vi "Meas Result Generate TWM Digitizer Correction.vi"(8 "error in":errorcluster, 11 "meas":T5={"swp cfg"={"N"=0, "R"=0, "f list"=[], "smpl delay"=0.0, "set delay"=0.0, "set delay np"=0.0, "meas root"=path "", "meas name"="", "meas a-index"=FALSE, "rnd sweep"=FALSE, "mode"=enum."Frequency", "swp mode"=enum."Linear", "avg"=0, "subrec"=0, "multi-freq"=FALSE, "selfcal"=FALSE, "selfcal period [h]"=0.0}, "bridge"={"type"=enum."TWM client", "TWM"={"pipe name"="", "parameters"=[], "handle"=0, "fixed aper [s]"=0.0, "f-list [Hz]"=[], "discrete f-list"=FALSE, "unc mode"=enum."None", "unc mcc"=0, "unc first"=FALSE, "alg id"=enum."TWM-LowZ - Low Z measurement"}, "last f"=0.0, "bias comp"={"bias type"=enum."dummy", "VISA"="", "Enable"=FALSE, "channel qu"=[], "channel Uinit"=[]}, "sim mode"=enum."Generic RLC network", "channel idns"=[], "sim phases"=1}, "src"={"type"=enum."Tektronix AFG3101C", "afg"={"VISA"="", "const"=0.0, "gen DC"=FALSE, "ext ref"=FALSE}, "cDAQ dds"={"device"="", "channels"=[], "mclk source"="", "mclk [Hz]"=0.0, "fs [Hz]"=0.0, "block [s]"=0.0, "buf [s]"=0.0, "task"="", "cmd queue"=refnum, "proc ref"=refnum, "smpl clock out"="/cDAQ3/PFI0", "export smpl clock"=FALSE, "DC ofs [V]"=[], "timebase source"="", "timebase mode"=enum."Local", "dither"=enum."Disabled", "dither level"=0.0, "phase [rad]"=[]}, "gain [V/A]"=1.0, "F5xxx session"={"VISA"="", "mode"=enum."AC voltage", "Earth on"=FALSE, "Ext ref lock"=FALSE}, "t3awg"={"VISA"="", "use ext ref"=FALSE, "ext ref [Hz]"=0.0, "load Z"=enum."High Z", "ramdac max n"=0, "noise dither [V]"=0.0, "t3awg fs rules"=[], "channels"=0, "ramdac min n"=0}}, "results"=refnum, "dvm"={"type"=enum."Disabled", "F5790"={"VISA"="", "Input"=enum."input 1", "Digital filter restart"=enum."medium", "hi resolution"=enum."off", "Digital filter mode"=enum."off", "ext guard"=FALSE}}, "thermo"={"type"=enum."COMET Tx5xx (ethernet)", "comment"="", "tag"="", "refresh"=5.0, "IP"="", "port"=502, "VISA"="", "last readout"=timestamp(0 s since 1904-01-01), "TCP ref"=refnum, "VISA sess"="", "idn"="", "press"=0.0, "RH"=0.0, "temp"=0.0, "pres cor"=[], "RH cor"=[], "temp cor"=[], "try left"=0, "failed"=FALSE, "RTD set"=[], "RTD inv"=[], "range"=0.0, "net mode"=enum."MODBUS", "try fail"=enum."Stop trying - return NaN", "timeout [s]"=0.0, "max retries"=0, "sim t [deg]"=0.0, "status"=0}} {"thermo"."status" items=["ok", "retry", "failed"]; "thermo"."RTD inv" format="%.1f"; "thermo"."RTD set" format="%.1f"; "thermo"."temp cor" format="%.1f"; "thermo"."RH cor" format="%.1f"; "thermo"."pres cor" format="%.1f"; "thermo"."refresh" min=0.1 max=1000.0 format="%.2f"; "src"."t3awg"."t3awg fs rules"."fs-step [Hz]" format="%#_6p"; "src"."t3awg"."t3awg fs rules"."fs-max [Hz]" format="%#_6p"; "src"."t3awg"."t3awg fs rules"."for f0 <" format="%#_6p"; "src"."t3awg"."t3awg fs rules"."fs-min [Hz]" format="%#_6p"; "src"."cDAQ dds"."channels" min=0 step=1; "bridge"."TWM"."f-list [Hz]" format="%#_6p"; "swp cfg"."f list"."bias" format="%#_3p"; "swp cfg"."f list"."level" format="%#_3p"; "swp cfg"."f list"."fs [Hz]" format="%#_5p"; "swp cfg"."f list"."time [s]" format="%#_3p"; "swp cfg"."f list"."f/fs" format="%#_3p"; "swp cfg"."f list"."periods" format="%#_3f"; "swp cfg"."f list"."f [Hz]" format="%#_5p"}) -> (0 "error out":errorcluster)   [LabVIEW 2020]
doc: "Generates simple TWM digitizer correction from measured data."
uses:
  meas session.ctl
  Meas Sweep Config.ctl
  Meas Freq Info.ctl
  meas_swp_mode.ctl
  meas_sweep_flist_mode.ctl
  bridge/Bridge Session.ctl
  bridge/Bridge Type.ctl
  drivers/TWM client/TWM Session.ctl
  drivers/TWM client/TWM parameters.ctl
  drivers/TWM client/Meas Proc QWTB Uncertainty Mode.ctl
  bridge/Bridge Algorithm.ctl
  bridge/Bridge Bias Session.ctl
  bridge/Bridge Bias Type.ctl
  bridge/Bridge Sim Mode.ctl
  source/Source Session.ctl
  source/Source Type.ctl
  drivers/AFG3101C/AFG3101C Session.ctl
  drivers/cDAQ DDS/cDAQ DDS Session.ctl
  drivers/cDAQ DDS/cDAQ DDS Setup.ctl
  drivers/cDAQ DDS/cDAQ DDS Timebase Mode.ctl
  drivers/cDAQ DDS/cDAQ DDS Dither.ctl
  drivers/Fluke 5XXX/top_lev/F5xxx_session.ctl
  drivers/Fluke 5XXX/top_lev/F5xxx_output_mode.ctl
  drivers/T3AWG3K/toplevel/T3AWG Session.ctl
  drivers/T3AWG3K/toplevel/T3AWG Load Z.ctl
  drivers/T3AWG3K/toplevel/fgen_ramdac_fs_rules.ctl
  results/Meas Results Ref.ctl
  results/Meas Results.ctl
  bridge/Bridge Frequency Readings Data.ctl
  drivers/TWM client/Meas Proc QWTB Spectrum Data.ctl
  drivers/TWM client/TWM Phase Info.ctl
  dvm/dvm session.ctl
  dvm/dvm type.ctl
  drivers/Fluke 5790A/top_level/F5790 session.ctl
  thermo/thermo.ctl
  thermo/thermo_types.ctl
  thermo/Thermometer Fail Action.ctl
  results/Meas Results Correction Structuring Mode.ctl
  Meas Results TWM Digitizer Correction Data.ctl
  Meas Results TWM Correction Digitizer Type.ctl
  Meas Results TWM InpZ Correction Uncertainty Config.ctl
  drivers/T3AWG3K/Active Technologies AWG3000.lvlib
panel:
  in  "u(Gp) [S]":dbl
  in  "u(Cp) [%]":dbl
  in  "u(Gp) [%]":dbl
  in  "u(Cp) [F]":dbl
  out "alg id":T1 caption="bridge.TWM.alg id"
  in  "Digitizer type":T2=enum."HP3458A"
  in  "Estimate non-linearity":bool
  in  "btn exit":bool
  out "last path":path
  out "correction data":T3
  in  "Use aperture correction":bool=TRUE
  in  "Use time shift":bool=TRUE
  in  "Mode":T4
  in  "btn export":bool
  out "table":string[][](table) caption="Overview"
  # "Uncertainty:"
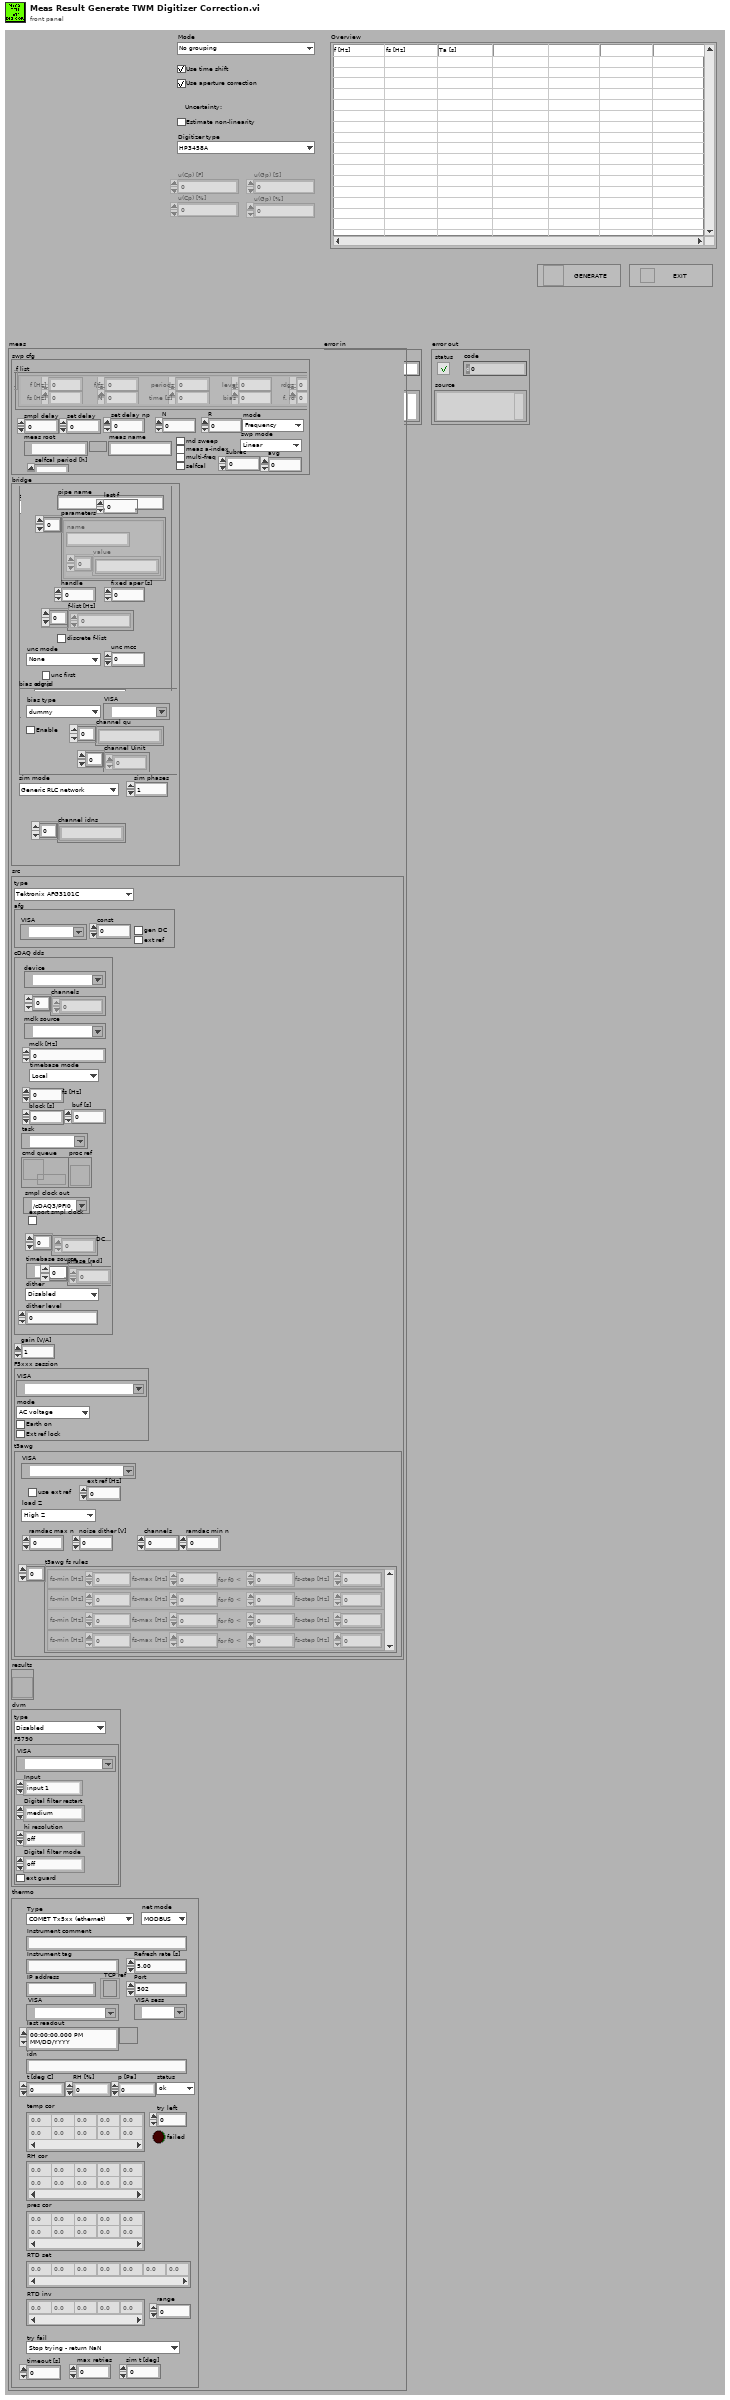
[diagram p1: front panel]
types:
  T1 = typedef "Bridge Algorithm.ctl" = enum16{"TWM-LowZ - Low Z measurement", "TWM-InpZ - Digitizer input Z measurement", "TWM-TIAZ - High Z using TIA"}
  T2 = typedef "Meas Results TWM Correction Digitizer Type.ctl" = enum16{"Unknown", "HP3458A", "NI9238"}
  T3 = typedef "Meas Results TWM Digitizer Correction Data.ctl" = cluster{"gains [V/V]":dbl[][][], "phases [rad]":dbl[][][], "timeshifts [s]":dbl[][], "f [Hz]":dbl[], "fs list [Hz]":dbl[], "aperture list [s]":dbl[], "channels":string[], "Mode":T4, "aperture correction":bool, "ranges [V]":dbl[], "amp [V]":dbl[][], "apertures [s]":dbl[], "unc gains [V/V]":dbl[][][], "unc phases [rad]":dbl[][][]}
  T4 = typedef "Meas Results Correction Structuring Mode.ctl" = enum16{"No grouping", "Group by apertures (3458A)", "Group by fs (generic digitizer)"}
  T5 = typedef "meas session.ctl" = cluster{"swp cfg":T6, "bridge":T10, "src":T18, "results":T29, "dvm":T30, "thermo":T33}
  T6 = typedef "Meas Sweep Config.ctl" = cluster{"N":i32, "R":i32, "f list":T7[], "smpl delay":dbl, "set delay":dbl, "set delay np":dbl, "meas root":path, "meas name":string, "meas a-index":bool, "rnd sweep":bool, "mode":T8, "swp mode":T9, "avg":i32, "subrec":i32, "multi-freq":bool, "selfcal":bool, "selfcal period [h]":dbl}
  T7 = typedef "Meas Freq Info.ctl" = cluster{"f [Hz]":dbl, "periods":dbl, "f/fs":dbl, "time [s]":dbl, "fs [Hz]":dbl, "N":i32, "level":dbl, "bias":dbl, "rdgs":i32, "f. id":i32}
  T8 = typedef "meas_swp_mode.ctl" = enum16{"Frequency", "Level", "Bias"}
  T9 = typedef "meas_sweep_flist_mode.ctl" = enum16{"Linear", "Log10"}
  T10 = typedef "Bridge Session.ctl" = cluster{"type":T11, "TWM":T12, "last f":dbl, "bias comp":T15, "sim mode":T17, "channel idns":string[], "sim phases":i32}
  T11 = typedef "Bridge Type.ctl" = enum16{"TWM client", "dummy"}
  T12 = typedef "TWM Session.ctl" = cluster{"pipe name":string, "parameters":T13[], "handle":i32, "fixed aper [s]":dbl, "f-list [Hz]":dbl[], "discrete f-list":bool, "unc mode":T14, "unc mcc":i32, "unc first":bool, "alg id":T1}
  T13 = typedef "TWM parameters.ctl" = cluster{"name":string, "value":string[]}
  T14 = typedef "Meas Proc QWTB Uncertainty Mode.ctl" = enum16{"None", "GUF", "Monte Carlo"}
  T15 = typedef "Bridge Bias Session.ctl" = cluster{"bias type":T16, "VISA":refnum<visa-resource-name>, "Enable":bool, "channel qu":string[], "channel Uinit":dbl[]}
  T16 = typedef "Bridge Bias Type.ctl" = enum16{"dummy", "CMI LiBbias V1.0"}
  T17 = typedef "Bridge Sim Mode.ctl" = enum16{"Generic RLC network", "Interchannel transfer", "Input impedance"}
  T18 = typedef "Source Session.ctl" = cluster{"type":T19, "afg":T20, "cDAQ dds":T21, "gain [V/A]":dbl, "F5xxx session":T24, "t3awg":T26}
  T19 = typedef "Source Type.ctl" = enum16{"Tektronix AFG3101C", "cDAQ DAC", "Fluke 5xxx", "Agilent 33120A", "R&S SMT", "Teledyne LeCroy T3AWG", "dummy"}
  T20 = typedef "AFG3101C Session.ctl" = cluster{"VISA":refnum<visa-resource-name>, "const":dbl, "gen DC":bool, "ext ref":bool}
  T21 = typedef "cDAQ DDS Session.ctl" = cluster{"device":tag, "channels":i32[], "mclk source":tag, "mclk [Hz]":dbl, "fs [Hz]":dbl, "block [s]":dbl, "buf [s]":dbl, "task":refnum<k21>, "cmd queue":refnum<queue>, "proc ref":refnum<vi>, "smpl clock out":tag, "export smpl clock":bool, "DC ofs [V]":dbl[], "timebase source":tag, "timebase mode":T22, "dither":T23, "dither level":dbl, "phase [rad]":dbl[]}
  T22 = typedef "cDAQ DDS Timebase Mode.ctl" = enum16{"Local", "Take from ADC (e.g. NI 9238)", "Other source"}
  T23 = typedef "cDAQ DDS Dither.ctl" = enum16{"Disabled", "Gaussian"}
  T24 = typedef "F5xxx_session.ctl" = cluster{"VISA":refnum<visa-resource-name>, "mode":T25, "Earth on":bool, "Ext ref lock":bool}
  T25 = typedef "F5xxx_output_mode.ctl" = enum16{"AC voltage", "AC current"}
  T26 = typedef "Active Technologies AWG3000.lvlib/T3AWG Session.ctl" = cluster{"VISA":refnum<visa-resource-name>, "use ext ref":bool, "ext ref [Hz]":dbl, "load Z":T27, "ramdac max n":i32, "noise dither [V]":dbl, "t3awg fs rules":T28[], "channels":i32, "ramdac min n":i32}
  T27 = typedef "Active Technologies AWG3000.lvlib/T3AWG Load Z.ctl" = enum16{"High Z", "50 Ohm"}
  T28 = typedef "Active Technologies AWG3000.lvlib/fgen_ramdac_fs_rules.ctl" = cluster{"fs-min [Hz]":dbl, "fs-max [Hz]":dbl, "for f0 < ":dbl, "fs-step [Hz]":dbl}
  T29 = typedef "Meas Results Ref.ctl" = refnum<vi>
  T30 = typedef "dvm session.ctl" = cluster{"type":T31, "F5790":T32}
  T31 = typedef "dvm type.ctl" = enum16{"Disabled", "Simulated", "Fluke 5790A"}
  T32 = typedef "F5790 session.ctl" = cluster{"VISA":refnum<visa-resource-name>, "Input":enum16{"input 1", "input 2", "wide-band"}, "Digital filter restart":enum16{"medium", "fine", "coarse"}, "hi resolution":enum16{"off", "on"}, "Digital filter mode":enum16{"off", "fast", "medium", "slow"}, "ext guard":bool}
  T33 = typedef "thermo.ctl" = cluster{"type":T34, "comment":string, "tag":string, "refresh":dbl, "IP":string, "port":u16, "VISA":refnum<visa-resource-name>, "last readout":timestamp, "TCP ref":refnum<k5>, "VISA sess":refnum<visa-resource-name>, "idn":string, "press":dbl, "RH":dbl, "temp":dbl, "pres cor":dbl[][], "RH cor":dbl[][], "temp cor":dbl[][], "try left":i32, "failed":bool, "RTD set":dbl[], "RTD inv":dbl[], "range":dbl, "net mode":enum16{"MODBUS", "HTTP"}, "try fail":T35, "timeout [s]":dbl, "max retries":i32, "sim t [deg]":dbl, "status":u16}
  T34 = typedef "thermo_types.ctl" = enum16{"Disabled", "Simulated", "COMET Tx5xx (ethernet)", "Keithley 2002 (GPIB) + RTD", "Agilent 344xx (GPIB) + RTD"}
  T35 = typedef "Thermometer Fail Action.ctl" = enum16{"Stop trying - keep last value", "Stop trying - return NaN", "Generate error - stop sweep"}
  T36 = typedef "Meas Results TWM InpZ Correction Uncertainty Config.ctl" = cluster{"u(Cp) [F]":dbl, "u(Cp) [%]":dbl, "u(Gp) [S]":dbl, "u(Gp) [%]":dbl}
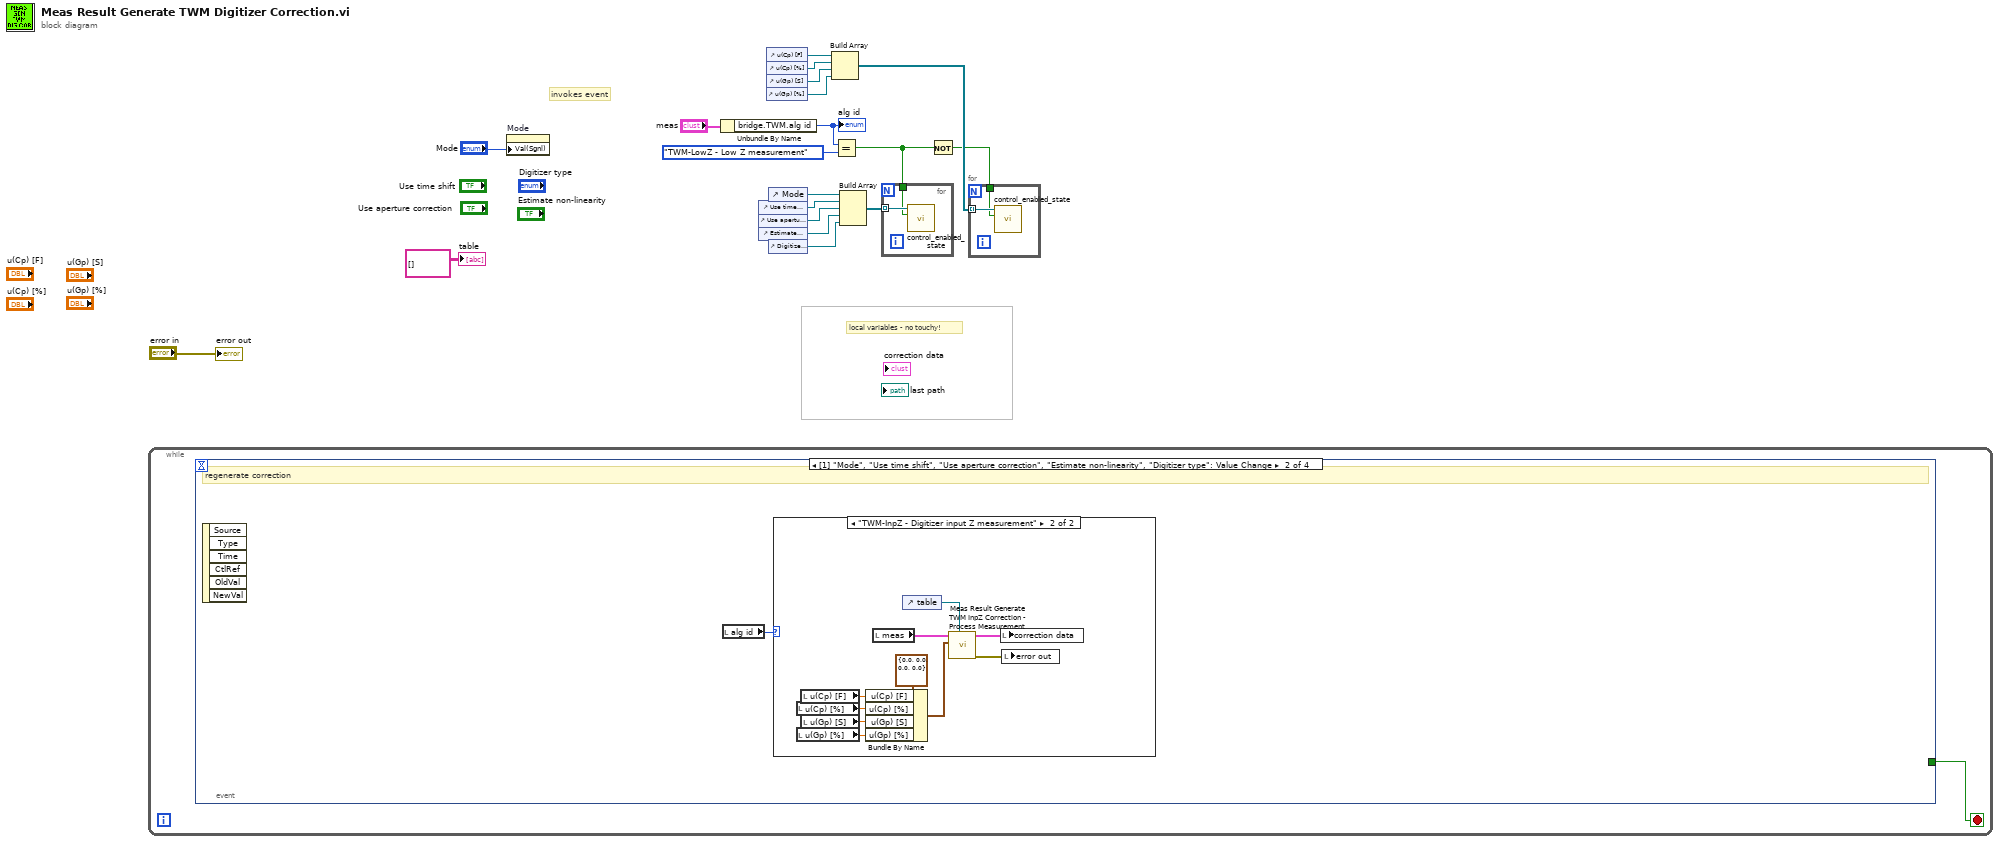
[diagram p0: block diagram]
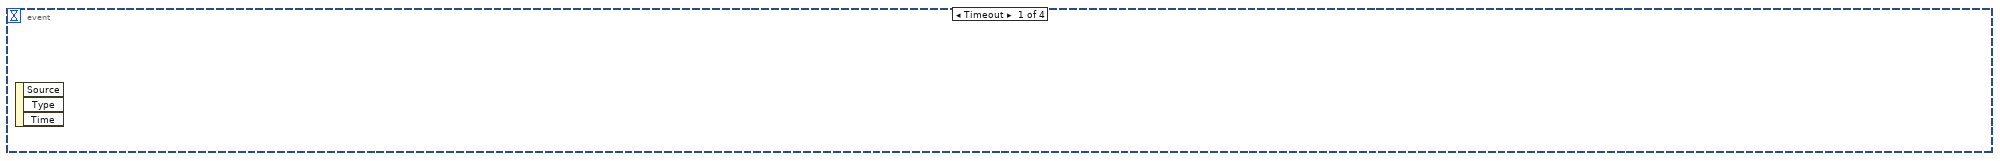
[diagram p2: hidden frame]
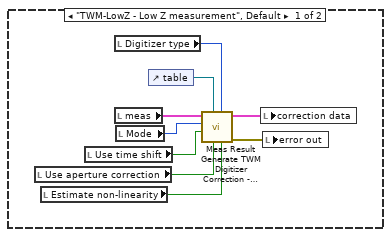
[diagram p3: hidden frame]
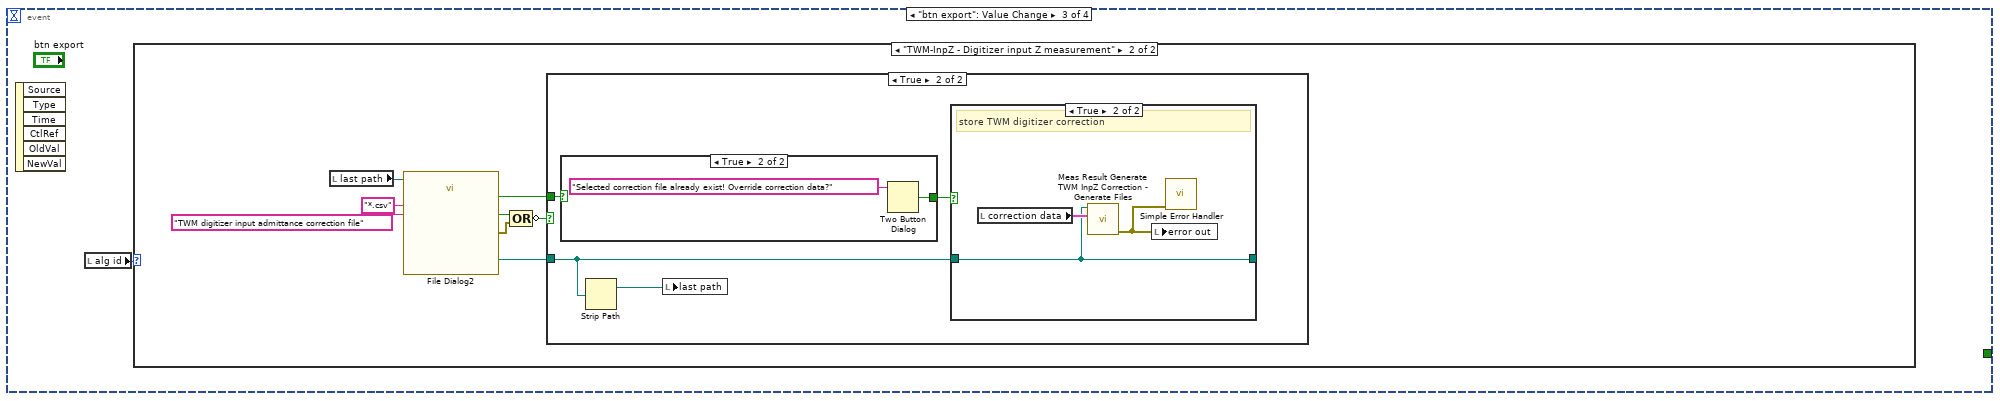
[diagram p4: hidden frame]
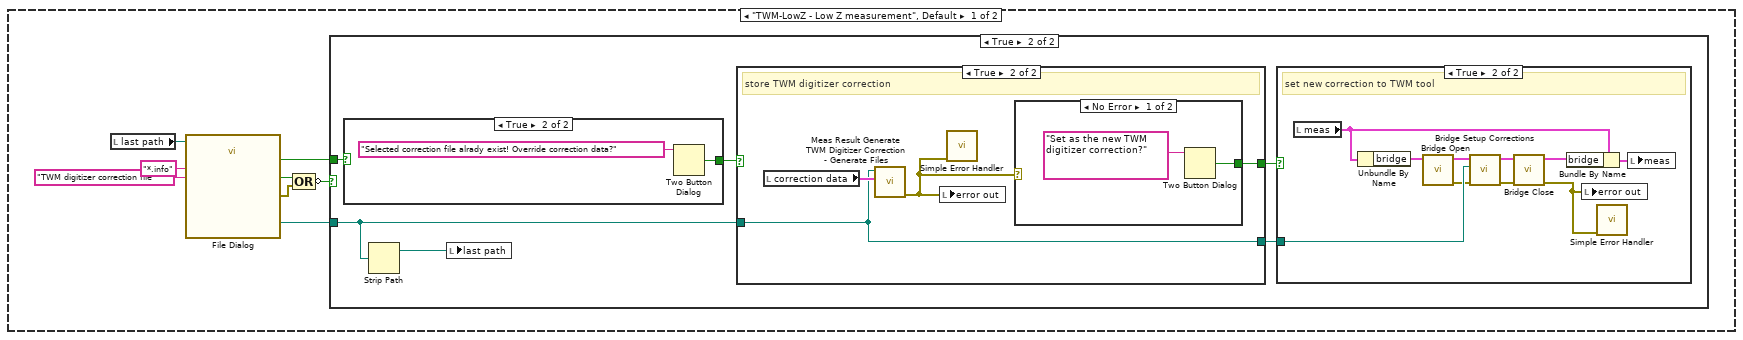
[diagram p5: hidden frame]
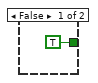
[diagram p8: hidden frame]
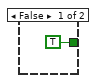
[diagram p12: hidden frame]
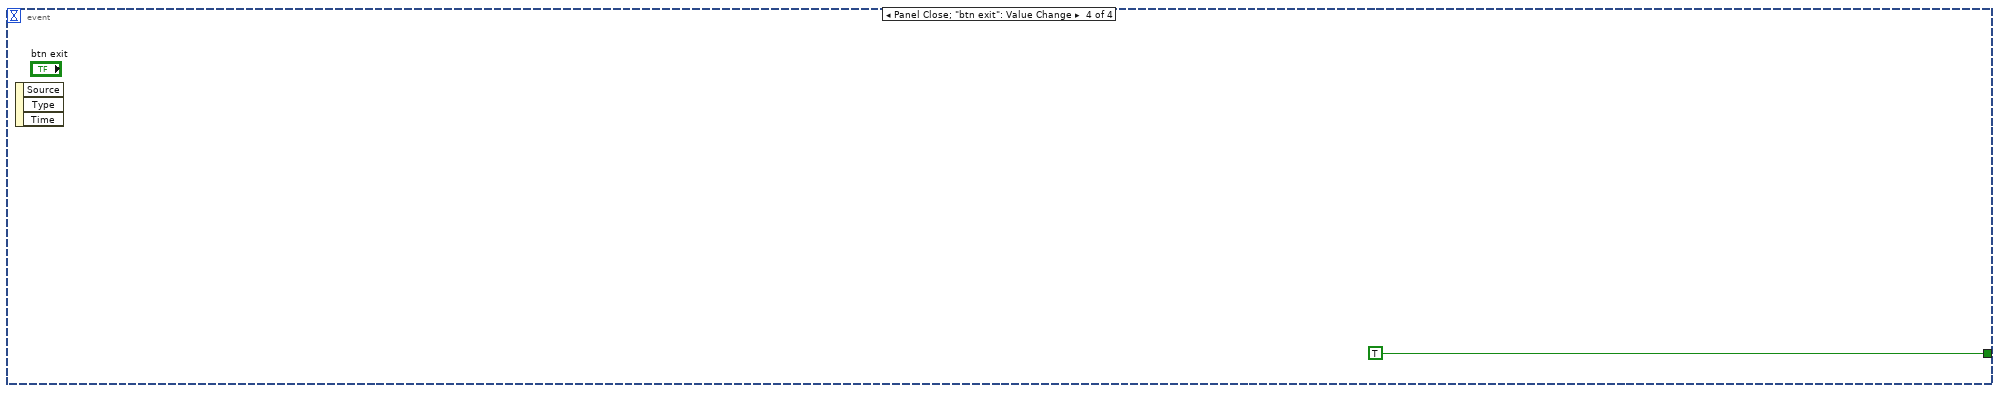
[diagram p14: hidden frame]
diagram:
  # "local variables - no touchy!"
  # "invokes event"
  n1 = while {
    stop <- w20 stop-if-true
    n2 = event shown="[1] \"Mode\", \"Use time shift\", \"Use aperture correction\", \"Estimate non-linearity\", \"Digitizer type\": Value Change" {
      selector: _ -> [_ _ _ _]
      dyn-events: _ -> [_ _ _ _]
      timeout: _ -> [_ _ _ _]
      tunnel: [_ _ _ TRUE] -> w20
      event Timeout {
        n3 = event-data() -> ()  [unwired: 1 in, 3 out]
      }
      event "Use time shift", "Use aperture correction", "Estimate non-linearity": Value Change {
        # "regenerate correction"
        n4 = event-data() -> ()  [unwired: 1 in, 6 out]
        n5 = local read "alg id"() -> (w21:T1)
        n6 = case shown="\"TWM-InpZ - Digitizer input Z measurement\"" w21 {
          frame "TWM-LowZ - Low Z measurement", Default {
            n7 = local read "Use aperture correction"() -> (w25:bool)
            n8 = local read "Estimate non-linearity"() -> (w23:bool)
            n9 = local read "Use time shift"() -> (w26:bool)
            n10 = local read "Digitizer type"() -> (w22:T2)
            n11 = local read "meas"() -> (w28:T5)
            n12 = local read "Mode"() -> (w27:T4)
            n13 = control-ref of="table"() -> (w29:refnum<vi>)
            n14 = call "Meas Result Generate TWM Digitizer Correction - Process Measurement.vi"("Estimate non-linearity (False)"=w23, "digitizer type"=w22, "use aperture correction (true)"=w25, "table ref"=w29, "use time shift (true)"=w26, "Mode"=w27, "meas"=w28) -> ("error out"=w30:errorcluster, "correction data"=w24:T3)  [unwired: 3 in]
            n15 = local write "correction data"(w24) -> ()
            n16 = local write "error out"(w30) -> ()
          }
          frame "TWM-InpZ - Digitizer input Z measurement" {
            n17 = local read "u(Cp) [%]"() -> (w33:dbl)
            n18 = local read "u(Gp) [%]"() -> (w36:dbl)
            n19 = local read "u(Cp) [F]"() -> (w34:dbl)
            n20 = local read "u(Gp) [S]"() -> (w35:dbl)
            n21 = Bundle By Name(cluster=T36 {"u(Cp) [F]"=0.0, "u(Cp) [%]"=0.0, "u(Gp) [S]"=0.0, "u(Gp) [%]"=0.0} ("inpz unc config"), "u(Cp) [F]"=w34, "u(Cp) [%]"=w33, "u(Gp) [S]"=w35, "u(Gp) [%]"=w36) -> (w31:T36)
            n22 = local read "meas"() -> (w38:T5)
            n23 = control-ref of="table"() -> (w39:refnum<vi>)
            n24 = call "Meas Result Generate TWM InpZ Correction - Process Measurement.vi"("table ref"=w39, "inpz unc config"=w31, "meas"=w38) -> ("error out"=w40:errorcluster, "correction data"=w37:T3)  [unwired: 7 in]
            n25 = local write "correction data"(w37) -> ()
            n26 = local write "error out"(w40) -> ()
          }
        }
      }
      event "btn export": Value Change {
        n27 = event-data() -> ()  [unwired: 1 in, 6 out]
        n28 = local read "alg id"() -> (w41:T1)
        n29 = case shown="\"TWM-InpZ - Digitizer input Z measurement\"" w41 {
          frame "TWM-LowZ - Low Z measurement", Default {
            n30 = local read "last path"() -> (w42:path)
            n31 = call "File Dialog"("start path"=w42, "pattern (all files)"="*.info", "pattern label"="TWM digitizer correction file") -> ("selected path"=w44:path, "exists"=w43:bool, "cancelled"=w47:bool, "error out"=w46:errorcluster)  [unwired: 9 in]
            n32 = Compound Arithmetic op=OR(w47, w46) -> (invert w45:bool)
            n33 = case shown="True" w45 {
              tunnel: w44 -> [_ w53]
              tunnel: w43 -> [_ w54]
              frame False {
              }
              frame True {
                n34 = case shown="True" w54 {
                  tunnel: [TRUE ("T button?") w67] -> w55
                  frame False {
                  }
                  frame True {
                    n35 = Two Button Dialog(message="Selected correction file alrady exist! Override correction data?") -> (T button?=w67:bool)  [unwired: 2 in]
                  }
                }
                n36 = Strip Path(path=w53) -> (stripped path=w52:path)  [unwired: 1 out]
                n37 = local write "last path"(w52) -> ()
                n38 = case shown="True" w55 {
                  tunnel: w53 -> [_ w69]
                  tunnel: [_ w70] -> w51
                  tunnel: [_ w69] -> w50
                  frame False {
                  }
                  frame True {
                    # "store TWM digitizer correction"
                    n39 = local read "correction data"() -> (w72:T3)
                    n40 = call "Meas Result Generate TWM Digitizer Correction - Generate Files.vi"("correction data"=w72, "correction root file"=w69) -> ("error out"=w71:errorcluster)  [unwired: 9 in]
                    n41 = local write "error out"(w71) -> ()
                    n42 = call <vilib>:"Simple Error Handler.vi"("error in (no error)"=w71) -> ()  [unwired: 4 in, 5 out]
                    n43 = case shown="No Error" w71 {
                      tunnel: [w73 _] -> w70
                      frame No Error {
                        n44 = Two Button Dialog(message="Set as the new TWM digitizer correction?") -> (T button?=w73:bool)  [unwired: 2 in]
                      }
                      frame Error {
                      }
                    }
                  }
                }
                n45 = case shown="True" w51 {
                  tunnel: w50 -> [_ w63]
                  frame False {
                  }
                  frame True {
                    # "set new correction to TWM tool"
                    n46 = local read "meas"() -> (w65:T5)
                    n47 = Unbundle By Name(w65) -> ("bridge"=w62:T10)
                    n48 = call "Bridge Open.vi"("bridge in"=w62) -> ("error out"=w60:errorcluster, "bridge out"=w61:T10)  [unwired: 7 in, 2 out]
                    n49 = call "Bridge Setup Corrections.vi"("error in"=w60, "digitizer correction path"=w63, "bridge in"=w61) -> ("error out"=w59:errorcluster, "bridge out"=w58:T10)  [unwired: 7 in]
                    n50 = call "Bridge Close.vi"("error in"=w59, "bridge in"=w58) -> ("error out"=w56:errorcluster, "bridge out"=w57:T10)  [unwired: 8 in]
                    n51 = Bundle By Name(cluster=w65, "bridge"=w57) -> (w64:T5)
                    n52 = local write "error out"(w56) -> ()
                    n53 = call <vilib>:"Simple Error Handler.vi"("error in (no error)"=w56) -> ()  [unwired: 4 in, 5 out]
                    n54 = local write "meas"(w64) -> ()
                  }
                }
              }
            }
          }
          frame "TWM-InpZ - Digitizer input Z measurement" {
            n55 = local read "last path"() -> (w75:path)
            n56 = call "File Dialog2"("start path"=w75, "pattern (all files)"="*.csv", "pattern label"="TWM digitizer input admittance correction file") -> ("selected path"=w77:path, "exists"=w76:bool, "cancelled"=w80:bool, "error out"=w79:errorcluster)  [unwired: 9 in]
            n57 = Compound Arithmetic op=OR(w80, w79) -> (invert w78:bool)
            n58 = case shown="True" w78 {
              tunnel: w77 -> [_ w84]
              tunnel: w76 -> [_ w85]
              frame False {
              }
              frame True {
                n59 = case shown="True" w85 {
                  tunnel: [TRUE ("T button?") w88] -> w86
                  frame False {
                  }
                  frame True {
                    n60 = Two Button Dialog(message="Selected correction file already exist! Override correction data?") -> (T button?=w88:bool)  [unwired: 2 in]
                  }
                }
                n61 = Strip Path(path=w84) -> (stripped path=w83:path)  [unwired: 1 out]
                n62 = local write "last path"(w83) -> ()
                n63 = case shown="True" w86 {
                  tunnel: w84 -> [_ w90]
                  tunnel: [_ w90] -> _
                  frame False {
                  }
                  frame True {
                    # "store TWM digitizer correction"
                    n64 = local read "correction data"() -> (w92:T3)
                    n65 = call "Meas Result Generate TWM InpZ Correction - Generate Files.vi"("correction data"=w92, "correction file path"=w90) -> ("error out"=w91:errorcluster)  [unwired: 9 in]
                    n66 = local write "error out"(w91) -> ()
                    n67 = call <vilib>:"Simple Error Handler.vi"("error in (no error)"=w91) -> ()  [unwired: 4 in, 5 out]
                  }
                }
              }
            }
          }
        }
      }
      event Panel Close; "btn exit": Value Change {
        n68 = event-data() -> ()  [unwired: 1 in, 3 out]
      }
    }
  }
  n69 = property on="Mode" class="Enum (strict)"("Val(Sgnl)"="Mode") -> ()  [unwired: 2 in, 2 out]
  n70 = Unbundle By Name("meas") -> ("bridge.TWM.alg id"=w9:T1)
  "alg id" <- w9
  n71 = control-ref of="Use time shift"() -> (w14:refnum<vi>)
  n72 = control-ref of="Use aperture correction"() -> (w13:refnum<vi>)
  n73 = control-ref of="Estimate non-linearity"() -> (w12:refnum<vi>)
  n74 = control-ref of="u(Cp) [F]"() -> (w7:refnum<vi>)
  n75 = control-ref of="u(Cp) [%]"() -> (w6:refnum<vi>)
  n76 = control-ref of="u(Gp) [S]"() -> (w5:refnum<vi>)
  n77 = control-ref of="u(Gp) [%]"() -> (w4:refnum<vi>)
  n78 = control-ref of="Mode"() -> (w15:refnum<vi>)
  n79 = control-ref of="Digitizer type"() -> (w11:refnum<vi>)
  n80 = Build Array(w7, w6, w5, w4) -> (w3:refnum<vi>[])
  n81 = Equal?(x=w9, y=Bridge_Algorithm."TWM-LowZ - Low Z measurement") -> (x = y?=w2:bool)
  n82 = Build Array(w15, w14, w13, w12, w11) -> (w10:refnum<vi>[])
  n83 = for {
    tunnel: w10 -> [w95] mode=indexing
    tunnel: w2 -> [w94]
    n84 = call "control_enabled_state.vi"("enabled"=w94, "control in"=w95) -> ()  [unwired: 6 in, 4 out]
  }
  n85 = Not(x=w2) -> (.not. x?=w1:bool)
  n86 = for {
    tunnel: w3 -> [w97] mode=indexing
    tunnel: w1 -> [w96]
    n87 = call "control_enabled_state.vi"("enabled"=w96, "control in"=w97) -> ()  [unwired: 6 in, 4 out]
  }
  "error out" <- "error in"
  "table" <- string[][] [] ("table")
